vi "_Calculate Next Value.vi"(0 "Iteration#":i32, 1 "Res Type":u8, 2 "# of Ramping Ch":u16, 3 "Parameter Offset":u16, 4 "Polarity":u8(ring) items=["Positive", "Negative", "Fast Scan"]) -> ()   [LabVIEW 2012]
uses:
  Type/_Table Type.ctl
  <vilib>/rvi/DataTransferAndStorage/Container/Common/niFpgaContainerGetUniqueNameForEmu.vi
  <vilib>/rvi/Memory/Memory_Emulation/niFpgaMemoryEmulationCacheClearOnFirstRun.vi
  <vilib>/rvi/Memory/Memory_Emulation/nirvimemoryEmulationManagerCache_MakeExclusive.vi
  <vilib>/rvi/Memory/Memory_Emulation/niFpgaMemoryEmulationValidateCache.vi
  <vilib>/rvi/Memory/Memory_Emulation/nirvimemoryEmulationManagerCache_ReleaseExclusive.vi
  <vilib>/rvi/Memory/Memory_Emulation/nirvimemoryEmulationManagerCache_InsertValue.vi
  <vilib>/Utility/error.llb/Clear Errors.vi
  <vilib>/rvi/Memory/Memory_Emulation/nirvimemoryEmulationManagerCache_GetValue.vi
  <vilib>/rvi/Emulation/niFpgaSctlEmulationGetInTimedLoop.vi
  <vilib>/rvi/Memory/Memory_Emulation/nirvimemoryEmulationManagerCache_SetValue.vi
  <vilib>/rvi/Emulation/niFpgaSctlEmulationResourceMgr.vi
  <vilib>/rvi/DataTransferAndStorage/Container/XNode/niFpgaContainer.xnode
  <vilib>/rvi/Memory/Memory_Emulation/nirvimemoryEmulation.vi
panel:
  # "Q1/Q2 Res Type:\n===========\n0  Hi/Hi\n1  Med/Med\n2  Lo/Lo\n3  Hi/Med\n4  Hi/Lo\n5  Med/Hi\n6  Med/Lo\n7  Lo/Hi\n8  Lo/Med"
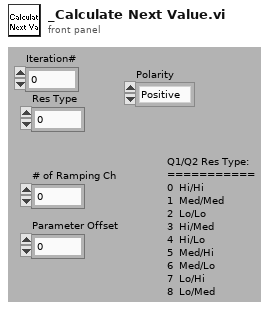
[diagram p1: front panel]
types:
  T1 = typedef "_Table Type.ctl" = enum8{"Q1 Cal +", "Q2 Cal +", "Q1 Cal -", "Q2 Cal -", "Q1 Res Hi +", "Q2 Res Hi +", "Q1 Res Med +", "Q2 Res Med +", "Q1 Res Lo +", "Q2 Res Lo +", "Q1 Res Hi -", "Q2 Res Hi -", "Q1 Res Med -", "Q2 Res Med -", "Q1 Res Lo -", "Q2 Res Lo -"}
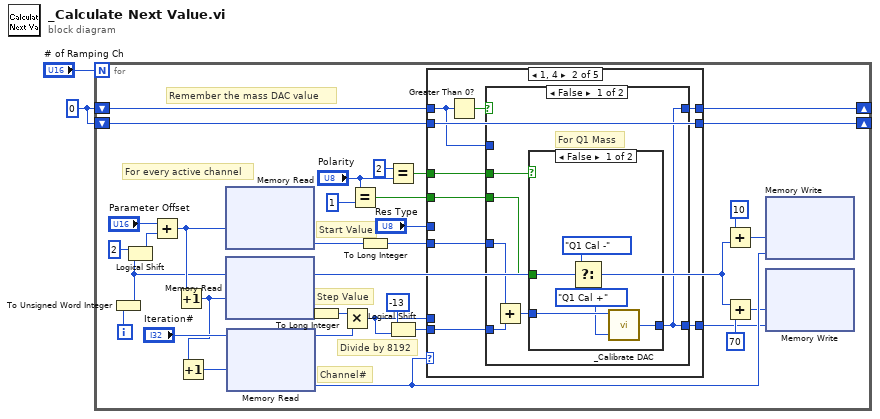
[diagram p0: block diagram]
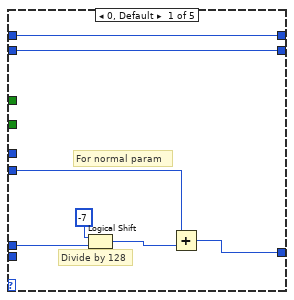
[diagram p2: hidden frame]
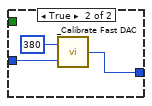
[diagram p3: hidden frame]
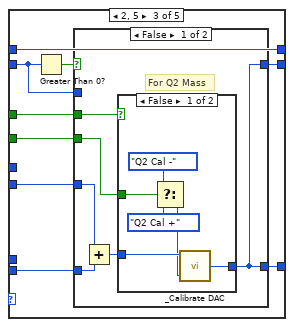
[diagram p5: hidden frame]
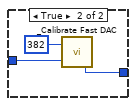
[diagram p6: hidden frame]
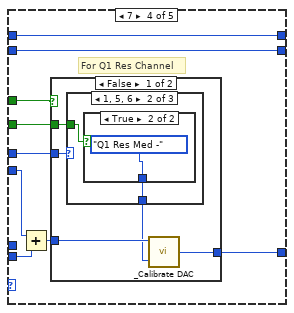
[diagram p8: hidden frame]
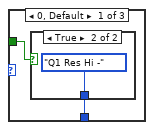
[diagram p9: hidden frame]
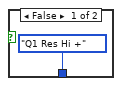
[diagram p10: hidden frame]
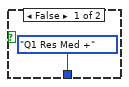
[diagram p11: hidden frame]
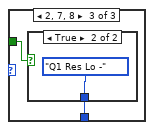
[diagram p12: hidden frame]
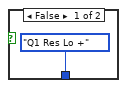
[diagram p13: hidden frame]
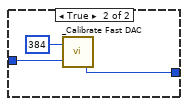
[diagram p14: hidden frame]
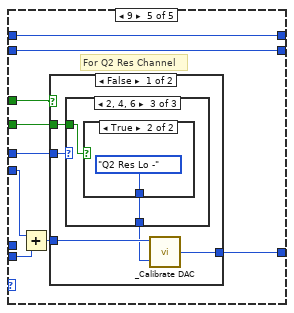
[diagram p15: hidden frame]
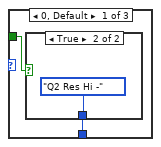
[diagram p16: hidden frame]
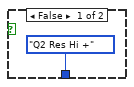
[diagram p17: hidden frame]
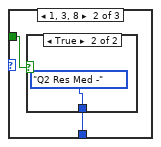
[diagram p18: hidden frame]
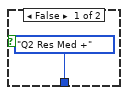
[diagram p19: hidden frame]
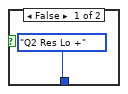
[diagram p20: hidden frame]
diagram:
  w1 = u32 0 ("y")
  n1 = for {
    N: "# of Ramping Ch" -> [_]
    shift-right: [w4] -> _
    shift-left: w1 -> [w6]
    shift-right: [w3] -> _
    shift-left: w1 -> [w5]
    i -> [w34]
    # "Remember the mass DAC value"
    # "Divide by 8192"
    # "Start Value"
    # "Channel#"
    # "Step Value"
    # "For every active channel"
    n2 = To Unsigned Word Integer(number=w34) -> (unsigned 16bit integer=w20:u16)
    n3 = Logical Shift(y=u16 2, x=w20) -> (x << y=w31:u16)
    n4 = Add(x="Parameter Offset", y=w31) -> (x+y=w25:u16)
    n5 = Increment(x=w25) -> (x+1=w21:u16)
    n6 = Increment(x=w21) -> (x+1=w22:u16)
    n7 = xnode ("Memory Read")("Address"=w25) -> ("Data"=w24:u32)  [unwired: 1 in, 1 out]
    n8 = xnode ("Memory Read")("Address"=w21) -> ("Data"=w23:u32)  [unwired: 1 in, 1 out]
    n9 = xnode ("Memory Read")("Address"=w22) -> ("Data"=w18:u32)  [unwired: 1 in, 1 out]
    n10 = To Long Integer(number=w23) -> (32bit integer=w30:i32)
    n11 = Multiply(x=w30, y="Iteration#") -> (x*y=w13:i32)
    n12 = Equal?(x="Polarity", y=u8 1) -> (x = y?=w10:bool)
    n13 = To Long Integer(number=w24) -> (32bit integer=w29:i32)
    n14 = Equal?(x=u8 2, y="Polarity") -> (x = y?=w7:bool)
    n15 = Logical Shift(y=-13, x=w13) -> (x << y=w12:i32)
    n16 = case shown="1, 4" w18 {
      tunnel: [w40 w50 w75 w98 w127] -> w16
      tunnel: w13 -> [w38 _ _ _ _]
      tunnel: w29 -> [w41 w49 w74 w100 w129]
      tunnel: "Res Type" -> [_ _ _ w97 w126]
      tunnel: w10 -> [_ w48 w73 w96 w125]
      tunnel: w12 -> [_ w47 w72 w95 w124]
      tunnel: w7 -> [_ w46 w71 w94 w123]
      tunnel: [w36 w42 w70 w93 w122] -> w4
      tunnel: w6 -> [w36 w43 w70 w93 w122]
      tunnel: [w35 w45 w67 w92 w121] -> w3
      tunnel: w5 -> [w35 w45 w68 w92 w121]
      frame 0, Default {
        # "Divide by 128"
        # "For normal param"
        n17 = Logical Shift(y=-7, x=w38) -> (x << y=w37:i32)
        n18 = Add(x=w41, y=w37) -> (x+y=w40:i32)
      }
      frame 1, 4 {
        n19 = Greater Than 0?(x=w43) -> (x > 0?=w44:bool)
        n20 = case shown="False" w44 {
          tunnel: [w51 w66] -> w50
          tunnel: w49 -> [w56 _]
          tunnel: w48 -> [w54 _]
          tunnel: w47 -> [w53 _]
          tunnel: w46 -> [w52 _]
          tunnel: w43 -> [_ w66]
          tunnel: [w51 w66] -> w42
          frame False {
            # "For Q1 Mass"
            n21 = Add(x=w56, y=w53) -> (x+y=w55:i32)
            n22 = case shown="False" w52 {
              tunnel: [w62 w63] -> w51
              tunnel: w55 -> [w61 w64]
              tunnel: w54 -> [w59 _]
              frame False {
                n23 = Select(t=_Table_Type."Q1 Cal -" ("Table Type"), s=w59, f=_Table_Type."Q1 Cal +" ("Table Type")) -> (s? t:f=w60:T1)
                n24 = call "_Calibrate DAC.vi"("Table Type"=w60, "Current Mass"=w61) -> ("DAC"=w62:u32)
              }
              frame True {
                n25 = call "_Calibrate Fast DAC.vi"("Mass (100x)"=w64, "Address"=u16 380) -> ("DAC"=w63:u32)
              }
            }
          }
          frame True {
          }
        }
      }
      frame 2, 5 {
        n26 = Greater Than 0?(x=w68) -> (x > 0?=w69:bool)
        n27 = case shown="False" w69 {
          tunnel: [w76 w91] -> w75
          tunnel: w74 -> [w81 _]
          tunnel: w73 -> [w79 _]
          tunnel: w72 -> [w78 _]
          tunnel: w71 -> [w77 _]
          tunnel: w68 -> [_ w91]
          tunnel: [w76 w91] -> w67
          frame False {
            # "For Q2 Mass"
            n28 = Add(x=w81, y=w78) -> (x+y=w80:i32)
            n29 = case shown="False" w77 {
              tunnel: [w87 w88] -> w76
              tunnel: w80 -> [w86 w89]
              tunnel: w79 -> [w85 _]
              frame False {
                n30 = Select(t=_Table_Type."Q2 Cal -" ("Table Type"), s=w85, f=_Table_Type."Q2 Cal +" ("Table Type")) -> (s? t:f=w82:T1)
                n31 = call "_Calibrate DAC.vi"("Table Type"=w82, "Current Mass"=w86) -> ("DAC"=w87:u32)
              }
              frame True {
                n32 = call "_Calibrate Fast DAC.vi"("Mass (100x)"=w89, "Address"=u16 382) -> ("DAC"=w88:u32)
              }
            }
          }
          frame True {
          }
        }
      }
      frame 7 {
        # "For Q1 Res Channel"
        n33 = Add(x=w100, y=w95) -> (x+y=w99:i32)
        n34 = case shown="False" w94 {
          tunnel: w99 -> [w105 w119]
          tunnel: [w104 w118] -> w98
          tunnel: w97 -> [w103 _]
          tunnel: w96 -> [w101 _]
          frame False {
            n35 = case shown="1, 5, 6" w103 {
              tunnel: [w107 w111 w115] -> w102
              tunnel: w101 -> [w106 w110 w114]
              frame 0, Default {
                n36 = case shown="True" w106 {
                  tunnel: [_Table_Type."Q1 Res Hi +" ("Table Type") _Table_Type."Q1 Res Hi -" ("Table Type")] -> w107
                  frame False {
                  }
                  frame True {
                  }
                }
              }
              frame 1, 5, 6 {
                n37 = case shown="True" w110 {
                  tunnel: [_Table_Type."Q1 Res Med +" ("Table Type") _Table_Type."Q1 Res Med -" ("Table Type")] -> w111
                  frame False {
                  }
                  frame True {
                  }
                }
              }
              frame 2, 7, 8 {
                n38 = case shown="True" w114 {
                  tunnel: [_Table_Type."Q1 Res Lo +" ("Table Type") _Table_Type."Q1 Res Lo -" ("Table Type")] -> w115
                  frame False {
                  }
                  frame True {
                  }
                }
              }
            }
            n39 = call "_Calibrate DAC.vi"("Table Type"=w102, "Current Mass"=w105) -> ("DAC"=w104:u32)
          }
          frame True {
            n40 = call "_Calibrate Fast DAC.vi"("Mass (100x)"=w119, "Address"=u16 384) -> ("DAC"=w118:u32)
          }
        }
      }
      frame 9 {
        # "For Q2 Res Channel"
        n41 = Add(x=w129, y=w124) -> (x+y=w128:i32)
        n42 = case shown="False" w123 {
          tunnel: w128 -> [w134 w148]
          tunnel: [w133 w147] -> w127
          tunnel: w126 -> [w132 _]
          tunnel: w125 -> [w130 _]
          frame False {
            n43 = case shown="2, 4, 6" w132 {
              tunnel: [w136 w140 w144] -> w131
              tunnel: w130 -> [w135 w139 w143]
              frame 0, Default {
                n44 = case shown="True" w135 {
                  tunnel: [_Table_Type."Q2 Res Hi +" ("Table Type") _Table_Type."Q2 Res Hi -" ("Table Type")] -> w136
                  frame False {
                  }
                  frame True {
                  }
                }
              }
              frame 1, 3, 8 {
                n45 = case shown="True" w139 {
                  tunnel: [_Table_Type."Q2 Res Med +" ("Table Type") _Table_Type."Q2 Res Med -" ("Table Type")] -> w140
                  frame False {
                  }
                  frame True {
                  }
                }
              }
              frame 2, 4, 6 {
                n46 = case shown="True" w143 {
                  tunnel: [_Table_Type."Q2 Res Lo +" ("Table Type") _Table_Type."Q2 Res Lo -" ("Table Type")] -> w144
                  frame False {
                  }
                  frame True {
                  }
                }
              }
            }
            n47 = call "_Calibrate DAC.vi"("Table Type"=w131, "Current Mass"=w134) -> ("DAC"=w133:u32)
          }
          frame True {
            n48 = call "_Calibrate Fast DAC.vi"("Mass (100x)"=w148, "Address"=u16 386) -> ("DAC"=w147:u32)
          }
        }
      }
    }
    n49 = Add(x=u16 10, y=w20) -> (x+y=w19:u16)
    n50 = Add(x=w20, y=u16 70 ("x")) -> (x+y=w17:u16)
    n51 = xnode ("Memory Write")("Address"=w19, "Data"=w18) -> ()  [unwired: 1 in, 1 out]
    n52 = xnode ("Memory Write")("Address"=w17, "Data"=w16) -> ()  [unwired: 1 in, 1 out]
  }
